vi "Updatable controls and indicators.vi"(8 "error in (no error)":errorcluster, 11 "PS Control Actor in":refnum<class "PS Control Actor.lvclass">) -> (0 "error out":errorcluster, 2 "Control type list":cluster{"Label":string, "Type":string}[](array[cluster])=[{"Label"="Field [T]", "Type"="d"}, {"Label"="Magnet Voltage", "Type"="d"}, {"Label"="Setpoint [T]", "Type"="d"}, {"Label"="Slew Rate [T/min]", "Type"="d"}, {"Label"="Status", "Type"="s"}], 3 "PS Control Actor out":refnum<class "PS Control Actor.lvclass">)   [LabVIEW 2019, in "PS Control Actor.lvlib" / "PS Control Actor.lvclass"]
uses:
  PS Control Actor.lvclass
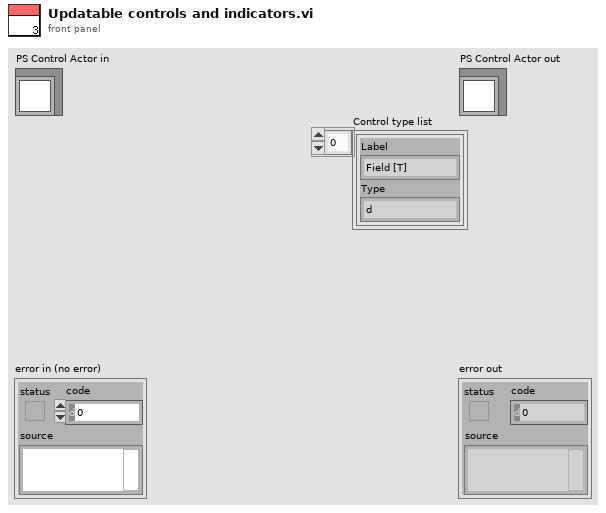
[diagram p1: front panel]
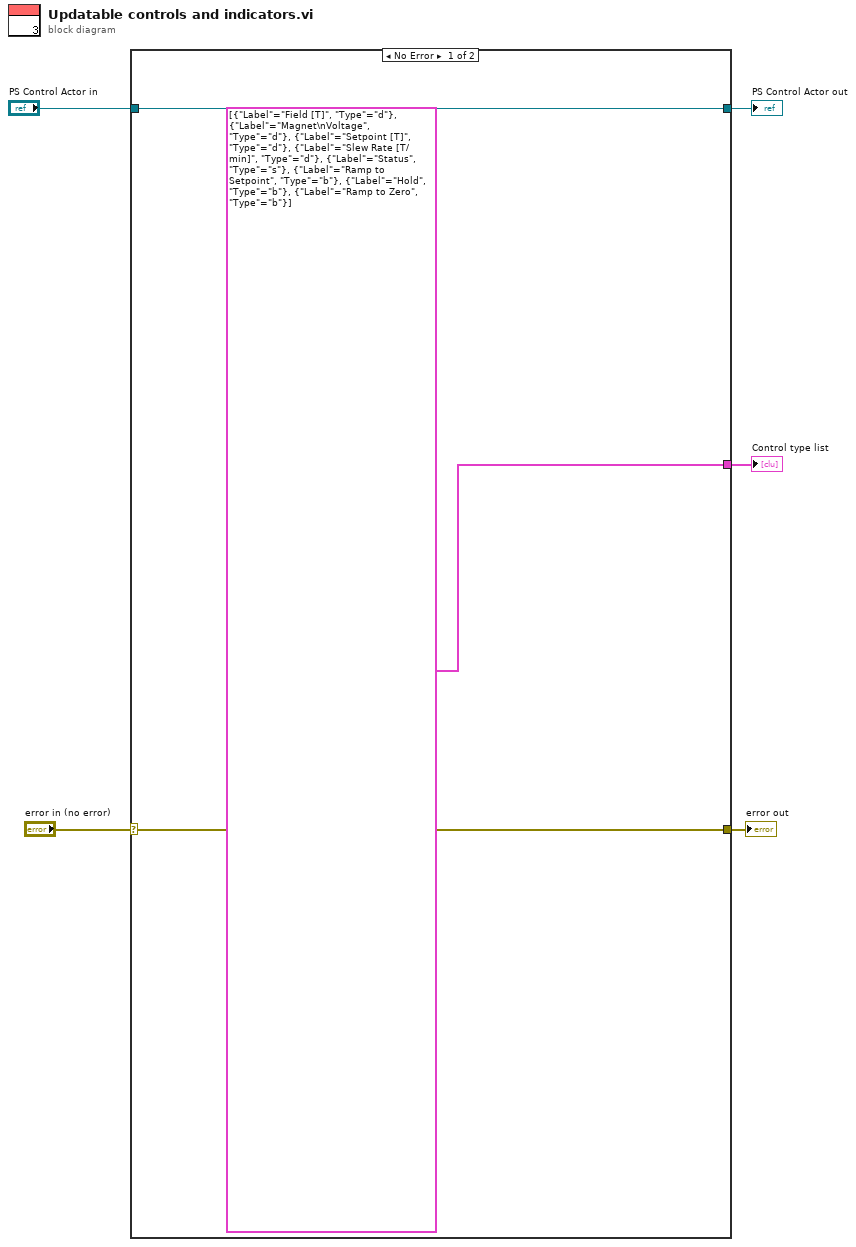
[diagram p0: block diagram]
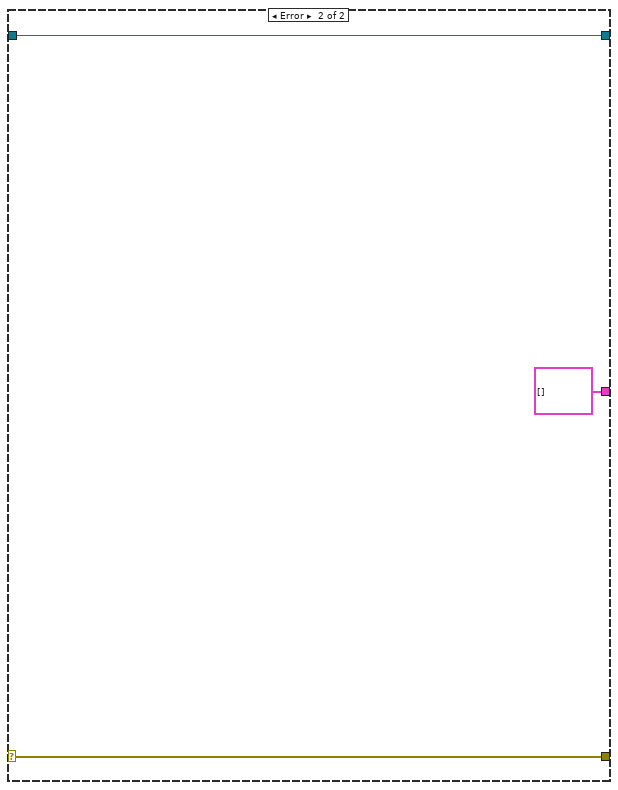
[diagram p2: hidden frame]
diagram:
  n1 = case shown="No Error" "error in (no error)" {
    selector: "error in (no error)" -> [w7 w11]
    tunnel: [w7 w11] -> w4
    tunnel: [w8 w10] -> w2
    tunnel: "PS Control Actor in" -> [w8 w10]
    tunnel: [cluster{"Label":string, "Type":string}[] [{"Label"="Field [T]", "Type"="d"}, {"Label"="Magnet\nVoltage", "Type"="d"}, {"Label"="Setpoint [T]", "Type"="d"}, {"Label"="Slew Rate [T/min]", "Type"="d"}, {"Label"="Status", "Type"="s"}, {"Label"="Ramp to Setpoint", "Type"="b"}, {"Label"="Hold", "Type"="b"}, {"Label"="Ramp to Zero", "Type"="b"}] ("Front panel controls") cluster{"Label":string, "Type":string}[] [] ("Front panel controls")] -> w1
    frame No Error {
    }
    frame Error {
    }
  }
  "error out" <- w4
  "PS Control Actor out" <- w2
  "Control type list" <- w1
